vi "prepare a b T.vi"(10 "par b":i32=1 min=1, 11 "par a":i32=1 min=1) -> (1 "T":i32, 2 "b":i32, 3 "a":i32)   [LabVIEW 2020]
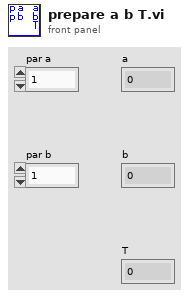
[diagram p1: front panel]
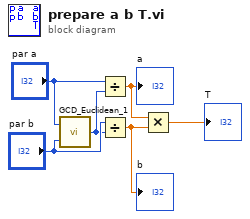
[diagram p0: block diagram]
diagram:
  n1 = call "GCD_Euclidean_1.vi"("integer 2"="par b", "integer 1"="par a") -> ("gcd"=w1:i32)
  n2 = Divide(x="par a", y=w1) -> (x/y=w4:dbl)
  "a" <- w4
  n3 = Divide(x="par b", y=w1) -> (x/y=w5:dbl)
  "b" <- w5
  n4 = Multiply(x=w4, y=w5) -> (x*y=→"T":dbl)
